vi "test1D Array Comparison.vi"(8 "error in (no error)":errorcluster, 11 "TestCase in":refnum<class "VITAC Example Test Case.lvclass">) -> (0 "error out":errorcluster, 3 "TestCase out":refnum<class "VITAC Example Test Case.lvclass">)   [LabVIEW 2015, in "VITAC Example Test Case.lvclass"]
doc: "An example of the 1d array function."
uses:
  VITAC Example Test Case.lvclass
  <vilib>/addons/_JKI Toolkits/VI Tester/TestCase.llb/TestCase.lvclass
  <vilib>/Wiresmith Technology/VITAC (VI Tester Advanced Comparisons)/VITAC.lvlib
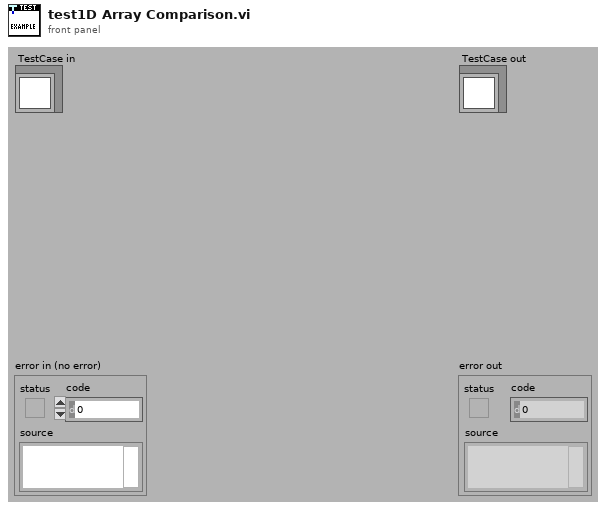
[diagram p1: front panel]
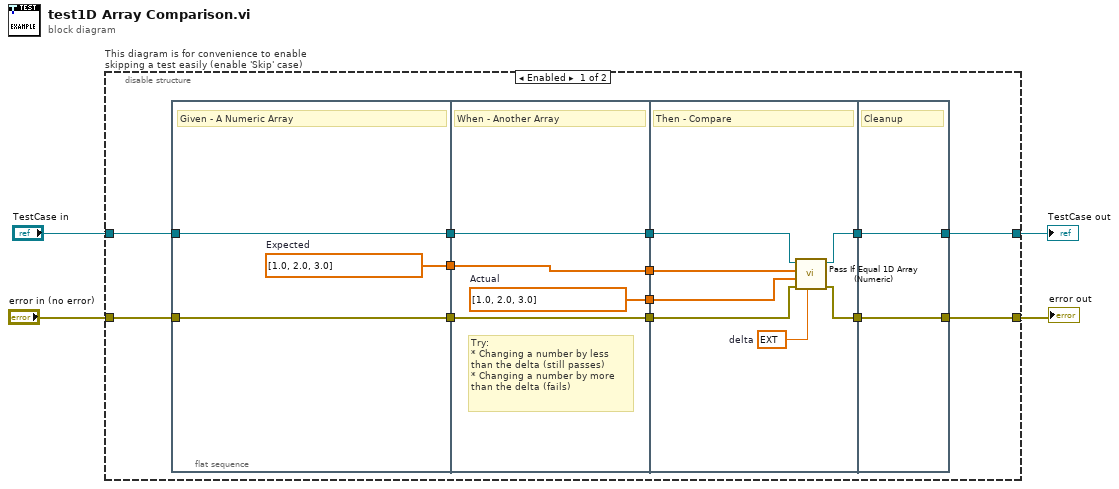
[diagram p0: block diagram]
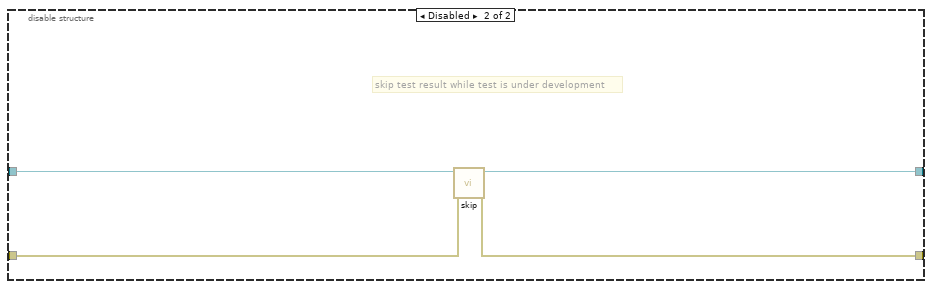
[diagram p2: hidden frame]
diagram:
  n1 = disable-structure "This diagram is for convenience to enable skipping a test easily (enable 'Skip' case)" shown="Enabled" {
    disable-tunnel: "TestCase in" -> [w11 w37]
    disable-tunnel: [w9 w35] -> w1
    disable-tunnel: [w8 w36] -> w3
    disable-tunnel: "error in (no error)" -> [w10 w34]
    frame Enabled {
      n2 = flat-sequence {
        tunnel: w10 -> [w19]
        tunnel: w11 -> [w20]
        tunnel: [w20] -> w17
        tunnel: [w19] -> w16
        tunnel: [w18] -> w7
        tunnel: [w24] -> w15
        tunnel: [w23] -> w14
        tunnel: w17 -> [w24]
        tunnel: w16 -> [w23]
        tunnel: w7 -> [w22]
        tunnel: [w22] -> w6
        tunnel: [w21] -> w5
        tunnel: [w30] -> w13
        tunnel: [w28] -> w12
        tunnel: w15 -> [w31]
        tunnel: w14 -> [w29]
        tunnel: w6 -> [w27]
        tunnel: w5 -> [w26]
        tunnel: [w32] -> w8
        tunnel: [w33] -> w9
        tunnel: w13 -> [w33]
        tunnel: w12 -> [w32]
        frame #0 {
          w18 = dbl[] [1.0, 2.0, 3.0]  # Expected
          # "Given - A Numeric Array"
        }
        frame #1 {
          w21 = dbl[] [1.0, 2.0, 3.0]  # Actual
          # "Try:\n* Changing a number by less \nthan the delta (still passes)\n* Changing a number by more\nthan the delta (fails)"
          # "When - Another Array"
        }
        frame #2 {
          w25 = ext 0.00000100000000000000000004  # delta
          # "Then - Compare"
          n3 = call <vilib>:"Pass If Equal 1D Array (Numeric).vi"("delta (optional)"=w25, "error in (no error)"=w29, "actual"=w26, "expected"=w27, "TestCase in"=w31) -> ("error out"=w28:errorcluster, "TestCase out"=w30:refnum<class "VITAC Example Test Case.lvclass">)  [unwired: 5 in]
        }
        frame #3 {
          # "Cleanup"
        }
      }
    }
    frame Disabled {
      # "skip test result while test is under development"
      n4 = call <vilib>:"skip.vi"("error in (no error)"=w34, "TestCase in"=w37) -> ("error out"=w36:errorcluster, "TestCase out"=w35:refnum<class "VITAC Example Test Case.lvclass">)  [unwired: 8 in]
    }
  }
  "error out" <- w3
  "TestCase out" <- w1
